vi "全局 提取仪器参数.vi"() -> ()   [LabVIEW 2016, in "数据传输系统-05.lvlib"]
panel:
  in  "参数编码":string
  in  "仪器编码":string
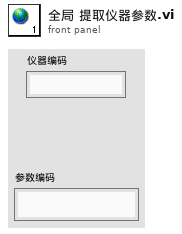
[diagram p1: front panel]
diagram:
